vi "CAlex2_SetCuff_Shank.vi"(6 "Reference Point":enum16{"Cuff Center", "Cuff Upper Edge"}(ring), 9 "ExtraWeight":dbl, 10 "Distance To Knee":dbl=0.15, 11 "Shank Length":dbl=0.42 format="%#_13g") -> (3 "Shank Cuff":T1={"BodyID"=0, "CoM(CuffCS)"={"Coord4"=[0.0, 0.0, 0.0, 1.0], "ID"=0}, "Mass(kg)"=0.0, "CablePts(CuffCS)"=[], "Cuff->Body"=[[1.0, 0.0, 0.0, 0.0], [0.0, 1.0, 0.0, 0.0], [0.0, 0.0, 1.0, 0.0], [0.0, 0.0, 0.0, 1.0]]})   [LabVIEW 2015, in "CAlex2.lvclass"]
uses:
  CAlex2.lvclass
  SerialChain-Cable/TypeDef/Cuff.ctl
  SerialChain/PointOnBody.ctl
  <vilib>/Analysis/Matrix/Datatypes/RealMatrix.ctl
  <vilib>/Analysis/Matrix/NI_Matrix.lvlib
  SerialChain/SerialChain.lvclass
  SerialChain-Cable/SerialChain-Cable.lvclass
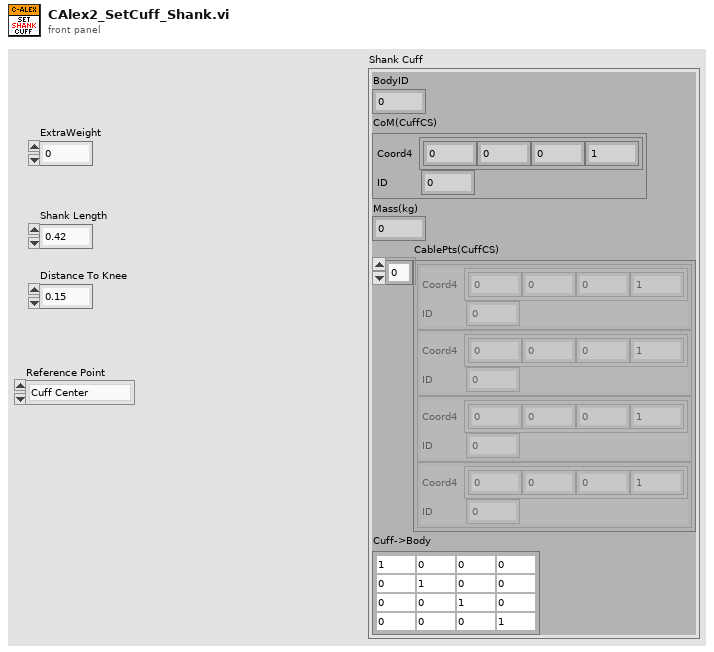
[diagram p1: front panel]
types:
  T1 = typedef "SerialChain-Cable.lvclass/Cuff.ctl" = cluster{"BodyID":i32, "CoM(CuffCS)":T2, "Mass(kg)":dbl, "CablePts(CuffCS)":T2[], "Cuff->Body":T3}
  T2 = typedef "SerialChain.lvclass/PointOnBody.ctl" = cluster{"Coord4":dbl[], "ID":i32}
  T3 = typedef "NI_Matrix.lvlib/RealMatrix.ctl" = dbl[][]
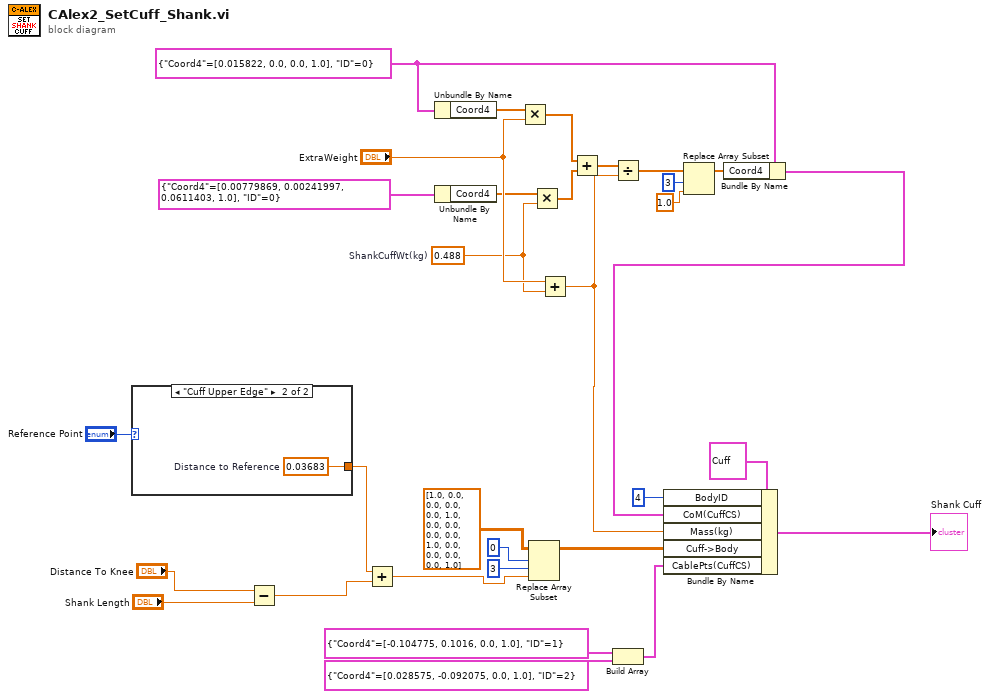
[diagram p0: block diagram]
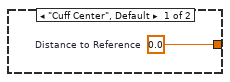
[diagram p2: hidden frame]
diagram:
  w9 = T2 {"Coord4"=[0.015822, 0.0, 0.0, 1.0], "ID"=0} ("CoM(CuffCS)")
  w1 = 0.488  # ShankCuffWt(kg)
  n1 = case shown="\"Cuff Upper Edge\"" "Reference Point" {
    tunnel: [w32 w33] -> w16
    frame "Cuff Center", Default {
      w32 = 0.0  # Distance to Reference
    }
    frame "Cuff Upper Edge" {
      w33 = 0.03683  # Distance to Reference
    }
  }
  n2 = Subtract(x="Distance To Knee", y="Shank Length") -> (x-y=w18:dbl)
  n3 = Add(x=w16, y=w18) -> (x+y=w17:dbl)
  n4 = Unbundle By Name(w9) -> ("Coord4"=w15:dbl[])
  n5 = Unbundle By Name(T2 {"Coord4"=[0.00779869, 0.00241997, 0.0611403, 1.0], "ID"=0} ("CoM(CuffCS)")) -> ("Coord4"=w13:dbl[])
  n6 = Multiply(x=w15, y="ExtraWeight") -> (x*y=w12:dbl[])
  n7 = Replace Array Subset(array=T3 [[1.0, 0.0, 0.0, 0.0], [0.0, 1.0, 0.0, 0.0], [0.0, 0.0, 1.0, 0.0], [0.0, 0.0, 0.0, 1.0]] ("Cuff->Leg"), new element=w17, index (row)=0, index (col)=3 ("index (row)")) -> (w28:T3)
  n8 = Multiply(x=w13, y=w1) -> (x*y=w11:dbl[])
  n9 = Add(x="ExtraWeight", y=w1) -> (x+y=w2:dbl)
  n10 = Add(x=w12, y=w11) -> (x+y=w10:dbl[])
  n11 = Divide(x=w10, y=w2) -> (x/y=w8:dbl[])
  n12 = Build Array(T2 {"Coord4"=[-0.104775, 0.1016, 0.0, 1.0], "ID"=1} ("CoM(CuffCS)"), T2 {"Coord4"=[0.028575, -0.092075, 0.0, 1.0], "ID"=2} ("CoM(CuffCS)")) -> (w27:T2[])
  n13 = Replace Array Subset(array=w8, new element=1.0 ("new element/subarray"), index=3) -> (w7:dbl[])
  n14 = Bundle By Name(cluster=w9, "Coord4"=w7) -> (w4:T2)
  n15 = Bundle By Name(cluster=T1 {"BodyID"=0, "CoM(CuffCS)"={"Coord4"=[0.0, 0.0, 0.0, 1.0], "ID"=0}, "Mass(kg)"=0.0, "CablePts(CuffCS)"=[], "Cuff->Body"=[[1.0, 0.0, 0.0, 0.0], [0.0, 1.0, 0.0, 0.0], [0.0, 0.0, 1.0, 0.0], [0.0, 0.0, 0.0, 1.0]]} ("Cuff Design"), "BodyID"=4, "CoM(CuffCS)"=w4, "Mass(kg)"=w2, "Cuff->Body"=w28, "CablePts(CuffCS)"=w27) -> (→"Shank Cuff":T1)
